vi "UTILITY JKI Loop Speed Adjust.vi"(4 "Current Rate":dbl, 5 "PID gains":T1={"proportional gain (Kc)"=0.1, "integral time (Ti, min)"=0.01, "derivative time (Td, min)"=0.0} {"derivative time (Td, min)" format="%.3f"; "integral time (Ti, min)" format="%.3f"; "proportional gain (Kc)" format="%.3f"}, 6 "Scan Rate Less Than 0.2s":bool, 7 "Use Fuzzy Logic":bool, 9 "K(7) - Adjustment Factor":dbl=0.3, 10 "Scan Rate Target":dbl, 11 "Previous Value":dbl) -> (3 "New Time":dbl)   [LabVIEW 2018]
panel:
  out "Going into Correction Loop?":bool
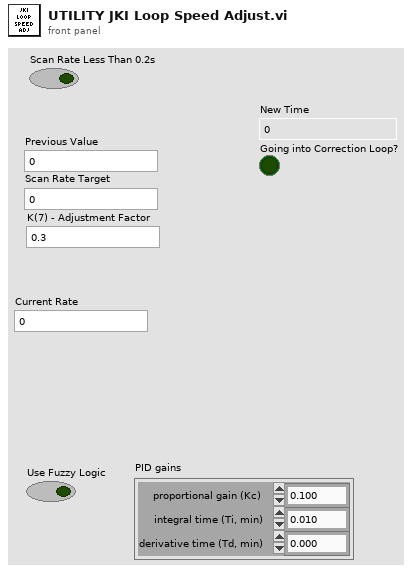
[diagram p1: front panel]
types:
  T1 = cluster{"proportional gain (Kc)":dbl, "integral time (Ti, min)":dbl, "derivative time (Td, min)":dbl}
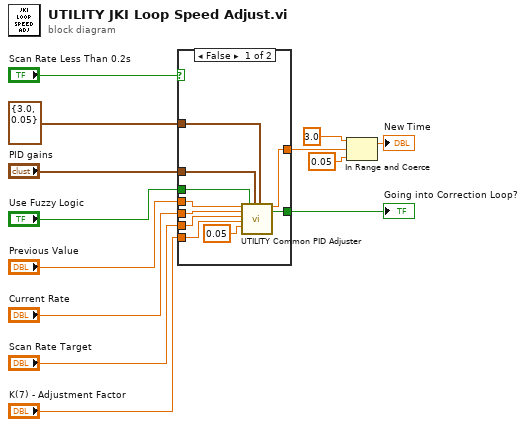
[diagram p0: block diagram]
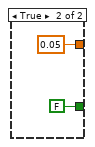
[diagram p2: hidden frame]
diagram:
  n1 = case shown="False" "Scan Rate Less Than 0.2s" {
    tunnel: [w23 0.05 ("New GPM Value")] -> w11
    tunnel: "Previous Value" -> [w22 _]
    tunnel: "Scan Rate Target" -> [w21 _]
    tunnel: "Current Rate" -> [w20 _]
    tunnel: "K(7) - Adjustment Factor" -> [w18 _]
    tunnel: [w17 FALSE ("Going into Correction Loop?")] -> w4
    tunnel: "Use Fuzzy Logic" -> [w16 _]
    tunnel: "PID gains" -> [w15 _]
    tunnel: cluster{"output high":dbl, "output low":dbl} {"output high"=3.0, "output low"=0.05} ("output range") -> [w14 _]
    frame False {
      n2 = call "UTILITY Common PID Adjuster.vi"("Previous Value"=w22, "Current Rate"=w20, "Scan Rate Target"=w21, "K(7) - Adjustment Factor"=w18, "ErrorPassBand(%)"=0.05, "Use Fuzzy Logic"=w16, "PID gains"=w15, "output range"=w14) -> ("New MicroAmp"=w23:dbl, "Going into Correction Loop?"=w17:bool)  [unwired: 8 in, 2 out]
    }
    frame True {
    }
  }
  "Going into Correction Loop?" <- w4
  n3 = In Range and Coerce(upper limit=3.0, x=w11, lower limit=0.05) -> (coerced(x)=→"New Time":dbl)  [unwired: 1 out]
